vi "Brightness Set.vi"(8 "error in (no error)":errorcluster, 11 "Enum":T1) -> (0 "error out":errorcluster)   [LabVIEW 2015]
uses:
  Brightness.ctl
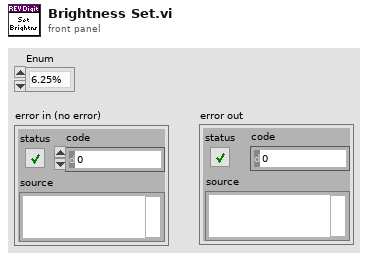
[diagram p1: front panel]
types:
  T1 = typedef "Brightness.ctl" = enum16{"6.25%", "12.5%", "18.75%", "25%", "31.25%", "37.5%", "43.74%", "50%", "56.25%", "62.5%", "68.75%", "75%", "81.25%", "87.5%", "93.75%", "100%"}
  T2 = typedef "WPI_I2CDevRef.ctl" = cluster{"DevStatus":errorcluster, "Device Address":u8, "Handle":i32, "I2C Bus":T3}
  T3 = typedef "i2c_bus.ctl" = enum16{"I2C On-Board", "I2C MXP", "Invalid"}
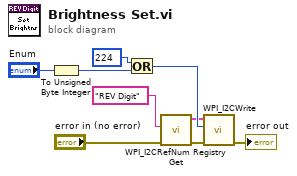
[diagram p0: block diagram]
diagram:
  n1 = To Unsigned Byte Integer(number="Enum") -> (unsigned 8bit integer=w8:u8)
  n2 = Or(x=u8 224 ("Device Address"), y=w8) -> (x .or. y?=w9:u8)
  n3 = call <vilib>:"WPI_I2CRefNum Registry Get.vi"("error in (no error)"="error in (no error)", "refnum name"="REV Digit") -> ("error out"=w1:errorcluster, "I2CDevRef"=w2:T2)  [unwired: 8 in]
  n4 = call <vilib>:"WPI_I2CWrite.vi"("error in (no error)"=w1, "I2CRegister"=w9, "I2CDevRef"=w2) -> ("error out"=→"error out":errorcluster)  [unwired: 7 in, 1 out]
